vi "UWB_Controller.vi"() -> ()   [LabVIEW 2016]
doc: "This VI controlls the DWM over UART. It starts of by resetting the DWM by sending a reset message over UART. It then starts sending CR messages to the DWM and poll for a response. When anything is received on the poll the DWM is operational. It then starts to request a position message which it saves in a global variable later used by the ROS publisher."
uses:
  <vilib>/myRIO/Instrument Drivers/Onboard IO/UART/typedef/VISA Configuration.ctl
  <vilib>/myRIO/Instrument Drivers/Onboard IO/DIO/typedefs/DIO Reference.ctl
  <vilib>/myRIO/Common/Instrument Driver Framework/Utilities/typedefs/myRIO Generic Hardware Reference.ctl
  <vilib>/myRIO/Common/Instrument Driver Framework/Utilities/typedefs/Hardware Version Enum.ctl
  <vilib>/myRIO/Common/Instrument Driver Framework/Utilities/typedefs/myRIO v1.0 Reference.ctl
  <vilib>/myRIO/Common/Instrument Driver Framework/Utilities/typedefs/Generic FPGA Reference.ctl
  <vilib>/myRIO/Common/Instrument Driver Framework/myRIO v1.0/DIO/typedefs/DIO Channels List.ctl
  <vilib>/myRIO/Common/Instrument Driver Framework/myRIO v1.0/DIO/typedefs/DIO Channels Enum.ctl
  <vilib>/userdefined/High Color/nirio_resource_hc.ctl
  <vilib>/myRIO/Common/Instrument Driver Framework/Utilities/vis/Is FPGA Ref Available.vi
  <vilib>/myRIO/Common/Instrument Driver Framework/roboRIO v1.0/DIO/vis/roboRIO v1.0 Open DIO.vi
  <vilib>/myRIO/Instrument Drivers/Onboard IO/DIO/vis/Write.vi
  <vilib>/myRIO/Common/Instrument Driver Framework/Utilities/vis/Validate Channels.vi
  <vilib>/myRIO/Common/Instrument Driver Framework/roboRIO v1.0/DIO/vis/roboRIO v1.0 Reserve DIO.vi
  <vilib>/myRIO/Common/Instrument Driver Framework/roboRIO v1.0/DIO/vis/roboRIO v1.0 Build MUX Configuration DIO.vi
  <vilib>/myRIO/Common/Instrument Driver Framework/roboRIO v1.0/Resource Manager/vis/roboRIO v1.0 Reserve Channel List.vi
  <vilib>/myRIO/Common/Instrument Driver Framework/roboRIO v1.0/Resource Manager/vis/roboRIO v1.0 Create Configuration List.vi
  <vilib>/myRIO/Common/Instrument Driver Framework/roboRIO v1.0/Resource Manager/vis/roboRIO v1.0 Reserve Channel.vi
  <vilib>/myRIO/Common/Instrument Driver Framework/roboRIO v1.0/Resource Manager/vis/roboRIO v1.0 Unreserve Channel.vi
  <vilib>/myRIO/Common/Instrument Driver Framework/roboRIO v1.0/Resource Manager/vis/roboRIO v1.0 Build Mutex Name.vi
  <vilib>/Instr/_visa.llb/VISA Configure Serial Port (Instr).vi
  GlobalVI.vi
  <vilib>/Utility/VariantDataType/GetNumericInfo.vi
  builds/UnicornMain/UnicornRIO1/ROS for LabVIEW/home/lvuser/natinst/bin/vi.lib/Utility/error.llb/Error Cluster From Error Code.vi
  <vilib>/myRIO/Common/Instrument Driver Framework/roboRIO v1.0/roboRIO v1.0 Open.vi
  <vilib>/myRIO/Common/Instrument Driver Framework/Utilities/vis/IO Manager.vi
  <vilib>/myRIO/Common/Instrument Driver Framework/Utilities/vis/Configuration Manager.vi
  <vilib>/myRIO/Common/Instrument Driver Framework/roboRIO v1.0/Resource Manager/vis/roboRIO v1.0 Configure IO.vi
  <vilib>/myRIO/Common/Instrument Driver Framework/myRIO v1.0/myRIO v1.0 Close.vi
  <vilib>/myRIO/Common/Instrument Driver Framework/roboRIO v1.0/DIO/vis/roboRIO v1.0 Write DIO.vi
  <vilib>/myRIO/Express VI/Onboard IO/UART/UART Express VI.xnode
  <vilib>/regexp/Match Regular Expression.xnode
  <vilib>/myRIO/Express VI/Onboard Devices/LED/LED Express VI.xnode
  <vilib>/myRIO/Instrument Drivers/Onboard IO/DIO/vis/myRIO DIO Open.xnode
  <vilib>/myRIO/Instrument Drivers/Onboard IO/UART/UART.lvlib
  <vilib>/myRIO/Instrument Drivers/Onboard IO/DIO/DIO.lvlib
panel:
  out "error out":errorcluster
  in  "error in OUTPUT 3":errorcluster
  in  "error in INPUT 2":errorcluster
  out "currentTimeout_Receive":u32
  out "error out OUTPUT 2":errorcluster
  out "offset past match\n(-1 = no match)":i32
  out "MSGFound":bool
  out "X":dbl
  out "Y":dbl
  out "Z":dbl
  out "error out INPUT":errorcluster
  out "timeoutError":bool
  out "currentTimeout":u32
  out "timeoutCount":u32
  out "timeoutValue":u32
  out "Resetting...":bool
  out "System ON":bool
  out "Receiving":bool
  out "Transmitting":bool
  out "UART Reset Buffer":string
  out "uwbState":i32
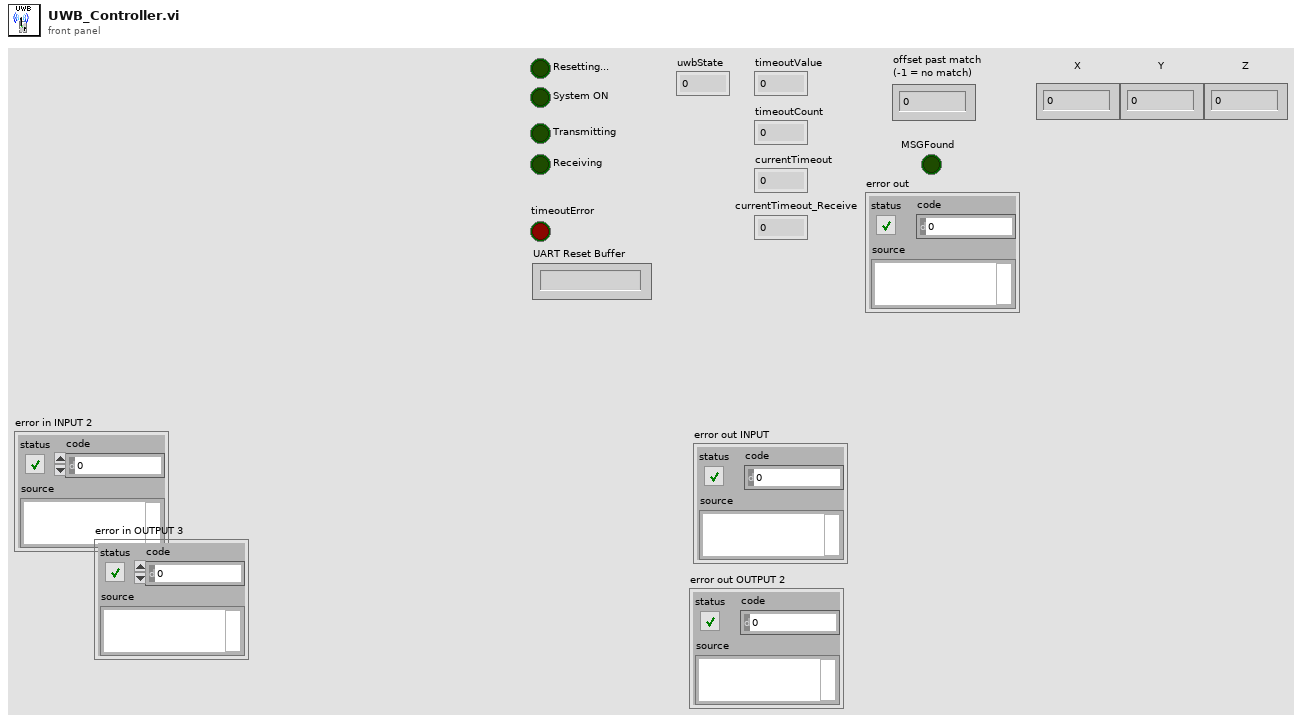
[diagram p1: front panel]
types:
  T1 = typedef "UART.lvlib/VISA Configuration.ctl" = cluster{"baud rate (9600)":u32, "data bits (8)":u16, "parity (0:none)":enum16{"None", "Odd", "Even", "Mark", "Space"}, "stop bits (10: 1 bit)":u16, "flow control (0:none)":u16, "termination char\n(0xA = '\\n' = LF) ":u8, "Enable Termination\nChar (T)":bool, "timeout (10sec)":u32}
  T2 = typedef "DIO.lvlib/DIO Reference.ctl" = cluster{"myRIO Reference":T3, "DIO Channels List":T7}
  T3 = typedef "myRIO Generic Hardware Reference.ctl" = cluster{"myRIO Model":T4, "myRIO Hardware Reference":T5}
  T4 = typedef "Hardware Version Enum.ctl" = enum16{"Unknown", "myRIO-1900", "myRIO-1950", "roboRIO", "NI ELVIS RIO CM"}
  T5 = typedef "myRIO v1.0 Reference.ctl" = cluster{"Generic FPGA Reference":T6, "Allow multiple opens":bool}
  T6 = typedef "Generic FPGA Reference.ctl" = refnum<k20>
  T7 = typedef "DIO Channels List.ctl" = T8[]
  T8 = typedef "DIO Channels Enum.ctl" = enum16{"Not Connected", "C/DIO0", "C/DIO1", "C/DIO2", "C/DIO3", "C/DIO4", "C/DIO5", "C/DIO6", "C/DIO7", "A/DIO0", "A/DIO1", "A/DIO2", "A/DIO3", "A/DIO4", "A/DIO5", "A/DIO6", "A/DIO7", "A/DIO8", "A/DIO9", "A/DIO10", "A/DIO11", "A/DIO12", "A/DIO13", "A/DIO14", "A/DIO15", "B/DIO0", "B/DIO1", "B/DIO2", "B/DIO3", "B/DIO4", "B/DIO5", "B/DIO6", "B/DIO7", "B/DIO8", "B/DIO9", "B/DIO10", "B/DIO11", "B/DIO12", "B/DIO13", "B/DIO14", "B/DIO15", "LED0", "LED1", "LED2", "LED3", "Button0", "DIO/DIO0", "DIO/DIO1", "DIO/DIO2", "DIO/DIO3", "DIO/DIO4", "DIO/DIO5", "DIO/DIO6", "DIO/DIO7", "DIO/DIO8", "DIO/DIO9", "SPI/CS0", "SPI/CS1", "SPI/CS2", "SPI/CS3", "LED RADIO (Green)", "LED RADIO (Red)", "LED COMM (Green)", "LED COMM (Red)", "LED MODE (Green)", "LED MODE (Red)"}
  T9 = typedef "nirio_resource_hc.ctl" = tag
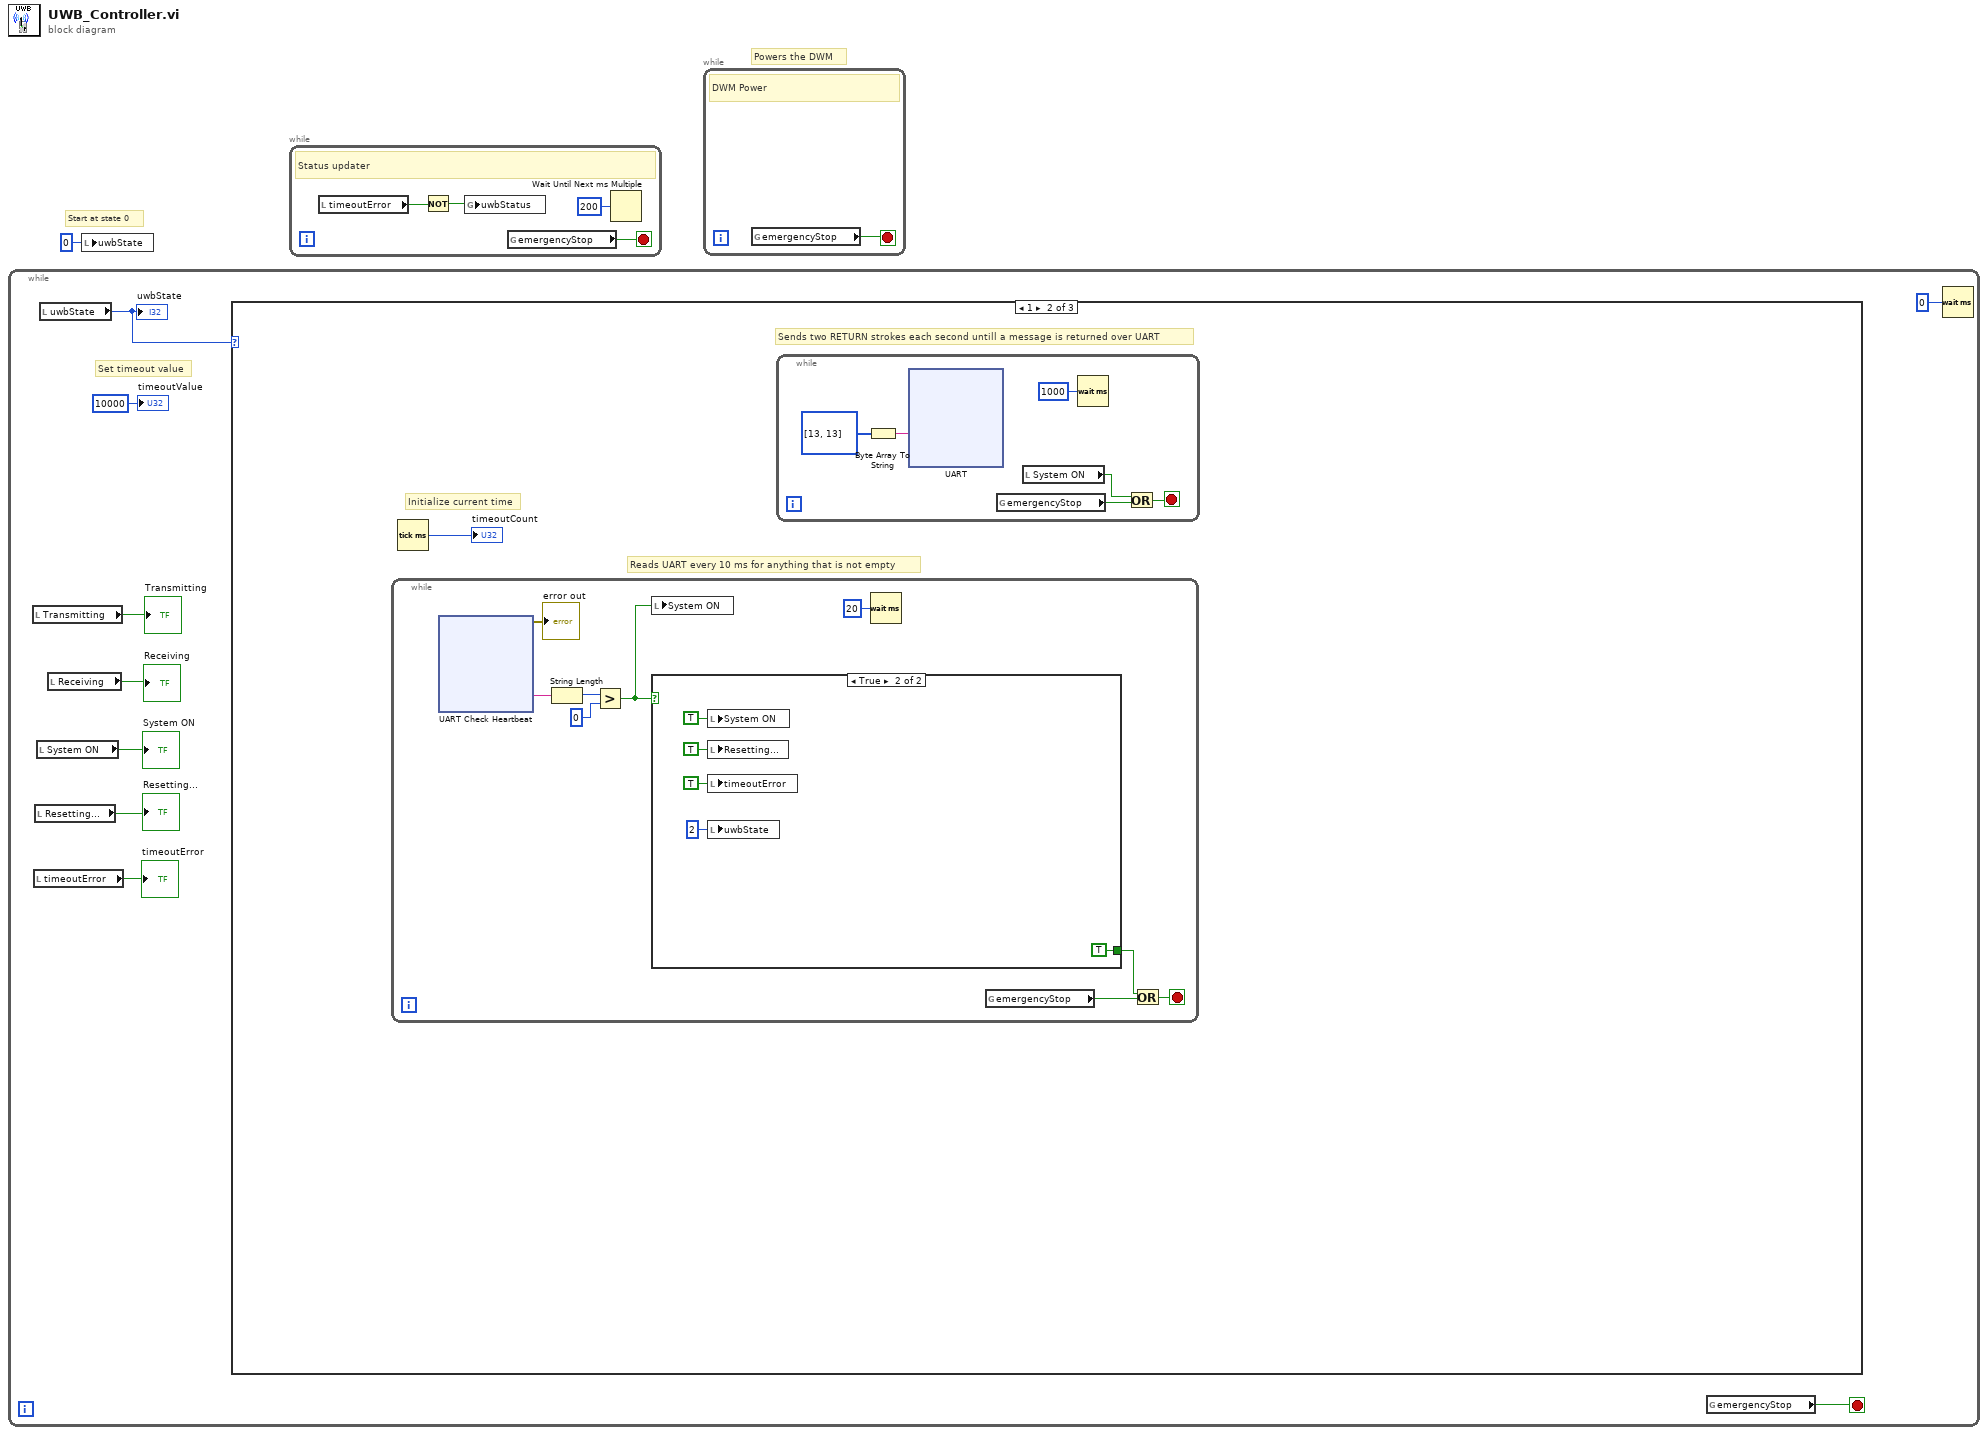
[diagram p0: block diagram]
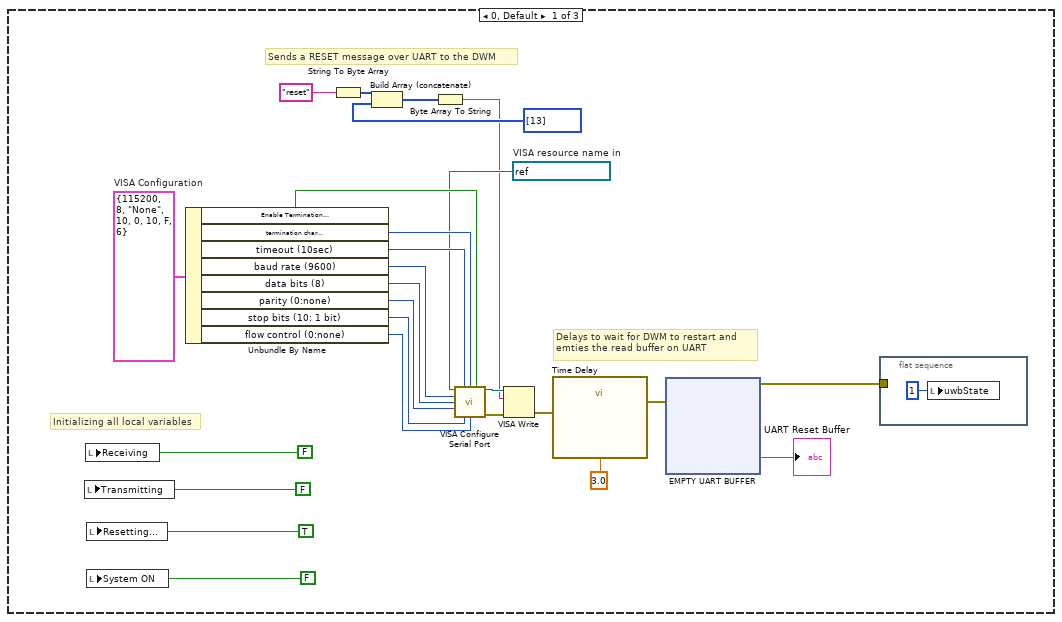
[diagram p2: hidden frame]
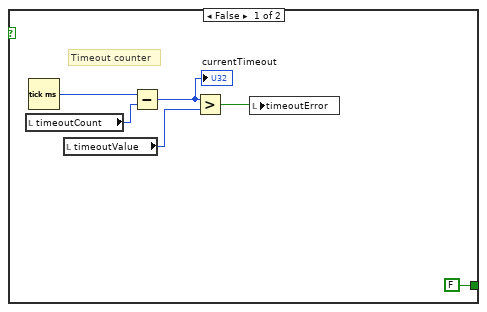
[diagram p3: hidden frame]
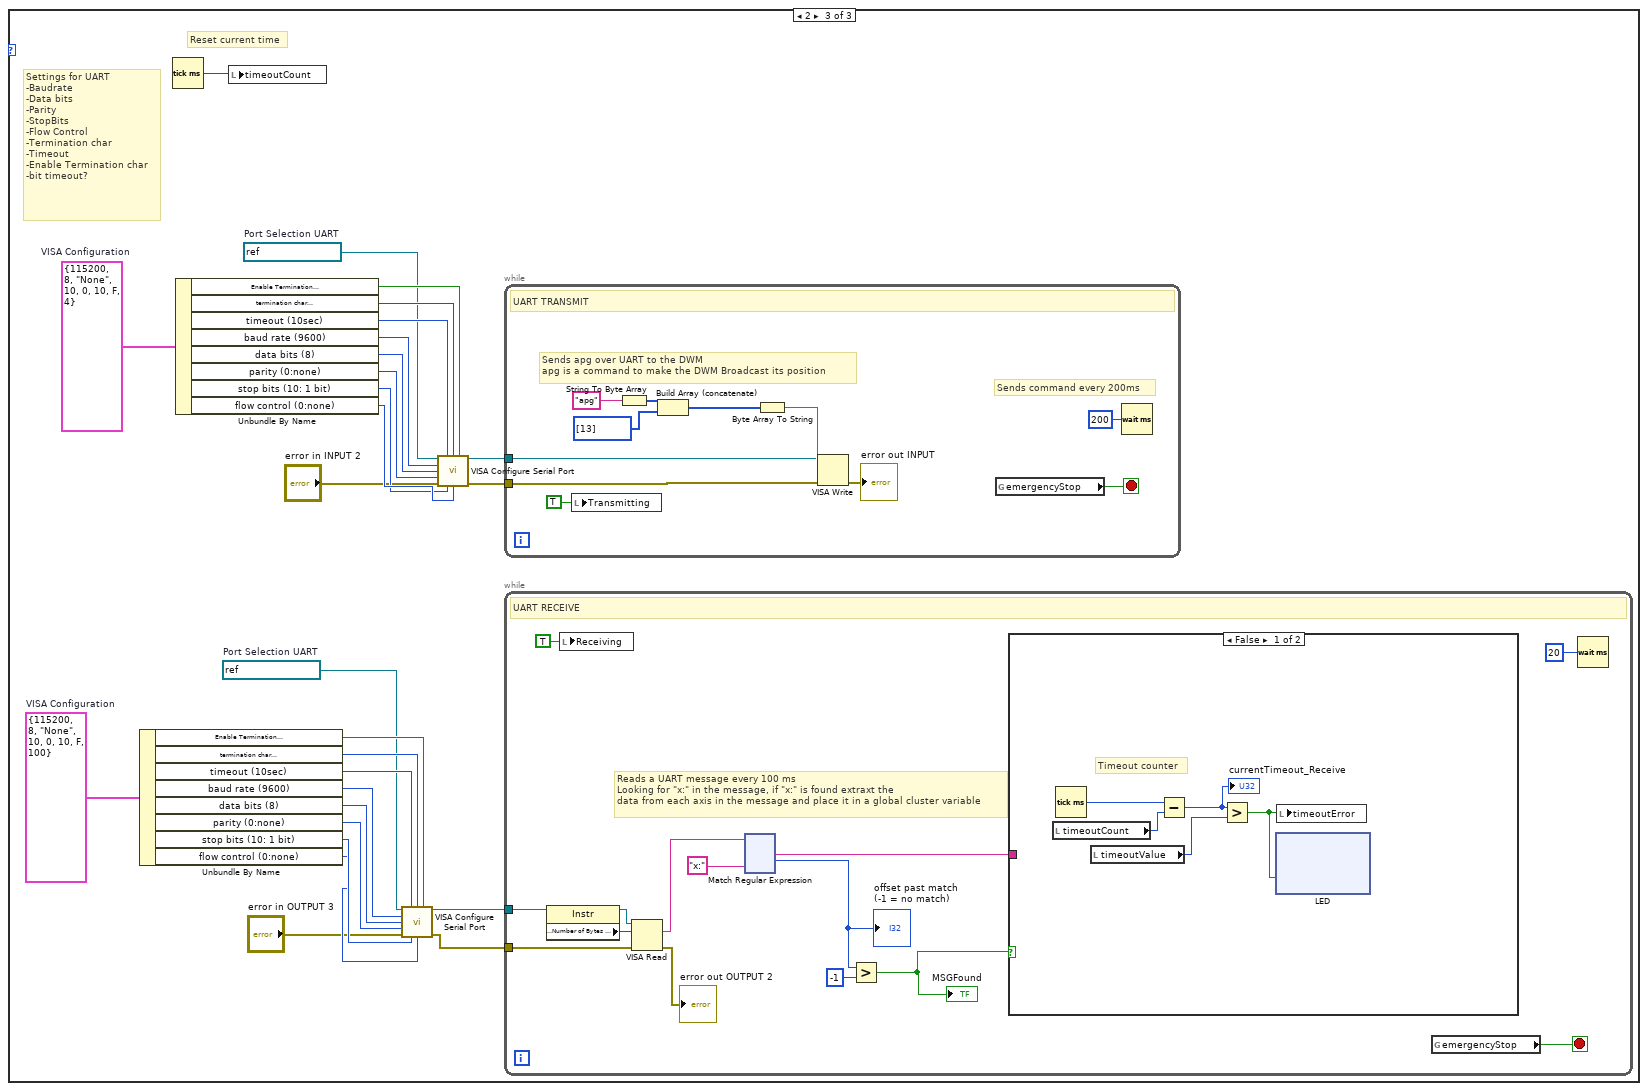
[diagram p4: hidden frame]
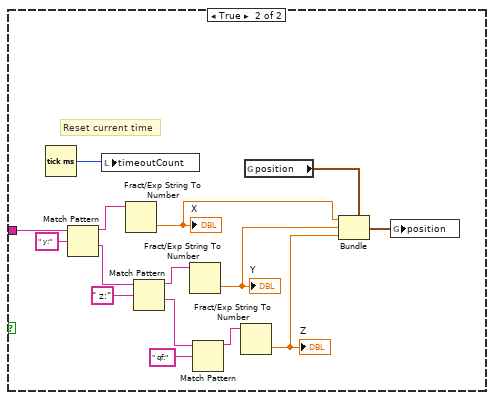
[diagram p5: hidden frame]
diagram:
  # "Powers the DWM"
  # "Start at state 0"
  n1 = while {
    stop <- w6 stop-if-true
    # "Set timeout value"
    n2 = local read "Transmitting"() -> (→"Transmitting":bool)
    n3 = local read "timeoutError"() -> (→"timeoutError":bool)
    n4 = local read "Resetting..."() -> (→"Resetting...":bool)
    n5 = local read "System ON"() -> (→"System ON":bool)
    n6 = local read "uwbState"() -> (w4:i32)
    "uwbState" <- w4
    n7 = local read "Receiving"() -> (→"Receiving":bool)
    n8 = case shown="1" w4 {
      frame 0, Default {
        w24 = T1 {"baud rate (9600)"=115200, "data bits (8)"=8, "parity (0:none)"=enum."None", "stop bits (10: 1 bit)"=10, "flow control (0:none)"=0, "termination char\n(0xA = '\\n' = LF) "=10, "Enable Termination\nChar (T)"=FALSE, "timeout (10sec)"=6}  # VISA Configuration
        w23 = refnum<visa-resource-name> "ASRL2::INSTR"  # VISA resource name in
        # "Initializing all local variables"
        # "Delays to wait for DWM to restart and \nemties the read buffer on UART"
        # "Sends a RESET message over UART to the DWM"
        n9 = local write "Transmitting"(FALSE ("Transmitting")) -> ()
        n10 = local write "Receiving"(FALSE ("Receiving")) -> ()
        n11 = local write "Resetting..."(TRUE ("Resetting...")) -> ()
        n12 = local write "System ON"(FALSE ("System On")) -> ()
        n13 = Unbundle By Name(w24) -> ("Enable Termination\nChar (T)"=w27:bool, "termination char\n(0xA = '\\n' = LF)"=w28:u8, "timeout (10sec)"=w29:u32, "baud rate (9600)"=w34:u32, "data bits (8)"=w33:u16, "parity (0:none)"=w32:enum16{"None", "Odd", "Even", "Mark", "Space"}, "stop bits (10: 1 bit)"=w31:u16, "flow control (0:none)"=w30:u16)
        n14 = String To Byte Array(string="reset") -> (unsigned byte array=w19:u8[])
        n15 = Build Array (concatenate)(w19, i32[] [13]) -> (w18:i32[])
        n16 = Byte Array To String(unsigned byte array=w18) -> (string=w17:string)
        n17 = call-poly "VISA Configure Serial Port"("VISA resource name"=w23, "timeout (10sec)"=w29, "termination char\n(0xA = '\\n' = LF)"=w28, "Enable Termination\nChar (T)"=w27, "baud rate (9600)"=w34, "data bits (8)"=w33, "parity (0:none)"=w32, "stop bits (10: 1 bit)"=w31, "flow control (0:none)"=w30) -> ("VISA resource name out"=w25:refnum<visa-resource-name>, "error out"=w26:errorcluster)  [unwired: 5 in]
        n18 = VISA Write(VISA resource name=w25, write buffer=w17, error in (no error)=w26) -> (error out=w22:errorcluster)  [unwired: 2 out]
        n19 = call "Time Delay"("error in (no error)"=w22, "Delay Time (s)"=3.0) -> ("error out"=w35:errorcluster)  [unwired: 9 in]
        n20 = xnode "EMPTY UART BUFFER"("error in (no error)"=w35) -> ("Characters Read"=→"UART Reset Buffer":string, "error out"=w11:errorcluster)
        n21 = flat-sequence {
          tunnel: w11 -> [_]
          frame #0 {
            n22 = local write "uwbState"(1 ("uwbState")) -> ()
          }
        }
      }
      frame 1 {
        # "Initialize current time"
        # "Reads UART every 10 ms for anything that is not empty"
        # "Sends two RETURN strokes each second untill a message is returned over UART"
        n23 = while {
          stop <- w81 stop-if-true
          n24 = xnode "UART Check Heartbeat"() -> ("Characters Read"=w86:string, "error out"=→"error out":errorcluster)  [unwired: 1 in]
          n25 = String Length(string=w86) -> (length=w85:i32)
          n26 = Greater?(x=w85, y=0) -> (0:w82:bool)
          n27 = local write "System ON"(w82) -> ()
          n28 = case shown="True" w82 {
            tunnel: [FALSE TRUE] -> w80
            frame False {
              # "Timeout counter"
              n29 = local read "timeoutCount"() -> (w89:u32)
              n30 = Tick Count (ms)() -> (millisecond timer value=w91:u32)
              n31 = local read "timeoutValue"() -> (w90:u32)
              n32 = Subtract(x=w91, y=w89) -> (x-y=w88:u32)
              "currentTimeout" <- w88
              n33 = Greater?(x=w88, y=w90) -> (0:w87:bool)
              n34 = local write "timeoutError"(w87) -> ()
            }
            frame True {
              n35 = local write "System ON"(TRUE ("System ON")) -> ()
              n36 = local write "Resetting..."(TRUE ("Resetting...")) -> ()
              n37 = local write "timeoutError"(TRUE ("timeoutError")) -> ()
              n38 = local write "uwbState"(2 ("uwbState")) -> ()
            }
          }
          n39 = Wait (ms)(milliseconds to wait=u32 20) -> ()  [unwired: 1 out]
          n40 = global read "GlobalVI.vi" "emergencyStop"() -> (w79:bool)
          n41 = Or(x=w80, y=w79) -> (x .or. y?=w81:bool)
        }
        n42 = Tick Count (ms)() -> (millisecond timer value=→"timeoutCount":u32)
        n43 = while {
          stop <- w57 stop-if-true
          n44 = Byte Array To String(unsigned byte array=u8[] [13, 13]) -> (string=w61:string)
          n45 = xnode "UART"("Characters to Write"=w61) -> ()  [unwired: 1 in, 2 out]
          n46 = global read "GlobalVI.vi" "emergencyStop"() -> (w58:bool)
          n47 = local read "System ON"() -> (w56:bool)
          n48 = Wait (ms)(milliseconds to wait=u32 1000) -> ()  [unwired: 1 out]
          n49 = Or(x=w56, y=w58) -> (x .or. y?=w57:bool)
        }
      }
      frame 2 {
        w118 = T1 {"baud rate (9600)"=115200, "data bits (8)"=8, "parity (0:none)"=enum."None", "stop bits (10: 1 bit)"=10, "flow control (0:none)"=0, "termination char\n(0xA = '\\n' = LF) "=10, "Enable Termination\nChar (T)"=FALSE, "timeout (10sec)"=100}  # VISA Configuration
        w117 = refnum<visa-resource-name> "ASRL2::INSTR"  # Port Selection UART
        w131 = T1 {"baud rate (9600)"=115200, "data bits (8)"=8, "parity (0:none)"=enum."None", "stop bits (10: 1 bit)"=10, "flow control (0:none)"=0, "termination char\n(0xA = '\\n' = LF) "=10, "Enable Termination\nChar (T)"=FALSE, "timeout (10sec)"=4}  # VISA Configuration
        w130 = refnum<visa-resource-name> "ASRL2::INSTR"  # Port Selection UART
        # "Settings for UART\n-Baudrate\n-Data bits\n-Parity\n-StopBits\n-Flow Control\n-Termination char\n-Timeout\n-Enable Termination char\n-bit timeout?"
        # "Reset current time"
        n50 = Unbundle By Name(w118) -> ("Enable Termination\nChar (T)"=w120:bool, "termination char\n(0xA = '\\n' = LF)"=w121:u8, "timeout (10sec)"=w122:u32, "baud rate (9600)"=w127:u32, "data bits (8)"=w126:u16, "parity (0:none)"=w125:enum16{"None", "Odd", "Even", "Mark", "Space"}, "stop bits (10: 1 bit)"=w124:u16, "flow control (0:none)"=w123:u16)
        n51 = Tick Count (ms)() -> (millisecond timer value=w141:u32)
        n52 = Unbundle By Name(w131) -> ("Enable Termination\nChar (T)"=w133:bool, "termination char\n(0xA = '\\n' = LF)"=w134:u8, "timeout (10sec)"=w135:u32, "baud rate (9600)"=w139:u32, "data bits (8)"=w138:u16, "parity (0:none)"=w137:enum16{"None", "Odd", "Even", "Mark", "Space"}, "stop bits (10: 1 bit)"=w136:u16, "flow control (0:none)"=w140:u16)
        n53 = local write "timeoutCount"(w141) -> ()
        n54 = call-poly "VISA Configure Serial Port"("VISA resource name"=w117, "timeout (10sec)"=w122, "termination char\n(0xA = '\\n' = LF)"=w121, "Enable Termination\nChar (T)"=w120, "baud rate (9600)"=w127, "data bits (8)"=w126, "parity (0:none)"=w125, "error in (no error)"="error in OUTPUT 3", "stop bits (10: 1 bit)"=w124, "flow control (0:none)"=w123) -> ("VISA resource name out"=w116:refnum<visa-resource-name>, "error out"=w115:errorcluster)  [unwired: 4 in]
        n55 = call-poly "VISA Configure Serial Port"("VISA resource name"=w130, "timeout (10sec)"=w135, "termination char\n(0xA = '\\n' = LF)"=w134, "Enable Termination\nChar (T)"=w133, "baud rate (9600)"=w139, "data bits (8)"=w138, "parity (0:none)"=w137, "error in (no error)"="error in INPUT 2", "stop bits (10: 1 bit)"=w136, "flow control (0:none)"=w140) -> ("VISA resource name out"=w129:refnum<visa-resource-name>, "error out"=w128:errorcluster)  [unwired: 4 in]
        n56 = while {
          tunnel: w129 -> [w326]
          tunnel: w128 -> [w325]
          stop <- w327 stop-if-true
          # "Sends command every 200ms"
          # "Sends apg over UART to the DWM\napg is a command to make the DWM Broadcast its position"
          # "UART TRANSMIT"
          n57 = local write "Transmitting"(TRUE ("Transmitting")) -> ()
          n58 = String To Byte Array(string="apg") -> (unsigned byte array=w332:u8[])
          n59 = Build Array (concatenate)(w332, i32[] [13]) -> (w331:i32[])
          n60 = Byte Array To String(unsigned byte array=w331) -> (string=w335:string)
          n61 = VISA Write(VISA resource name=w326, write buffer=w335, error in (no error)=w325) -> (error out=→"error out INPUT":errorcluster)  [unwired: 2 out]
          n62 = global read "GlobalVI.vi" "emergencyStop"() -> (w327:bool)
          n63 = Wait (ms)(milliseconds to wait=u32 200) -> ()  [unwired: 1 out]
        }
        n64 = while {
          tunnel: w116 -> [w143]
          tunnel: w115 -> [w142]
          stop <- w144 stop-if-true
          # "Reads a UART message every 100 ms\nLooking for \"x:\" in the message, if \"x:\" is found extraxt the\ndata from each axis in the message and place it in a global cluster variable"
          # "UART RECEIVE"
          n65 = property class="Instr"(reference=w143) -> (reference out=w153:refnum<visa-resource-name>, "Serial Settings:Number of Bytes at Serial Port"=w154:u32)  [unwired: 1 in, 1 out]
          n66 = local write "Receiving"(TRUE ("Receiving")) -> ()
          n67 = VISA Read(VISA resource name=w153, byte count=w154, error in (no error)=w142) -> (read buffer=w147:string, error out=→"error out OUTPUT 2":errorcluster)  [unwired: 2 out]
          n68 = xnode "Match Regular Expression"("input string"=w147, "regular expression"="x:") -> ("after match"=w146:string, "offset past match"=w150:i32)  [unwired: 4 in, 3 out]
          "offset past match\n(-1 = no match)" <- w150
          n69 = Greater?(x=w150, y=-1) -> (0:w148:bool)
          "MSGFound" <- w148
          n70 = case shown="False" w148 {
            tunnel: w146 -> [_ w202]
            frame False {
              # "Timeout counter"
              n71 = local read "timeoutCount"() -> (w158:u32)
              n72 = Tick Count (ms)() -> (millisecond timer value=w160:u32)
              n73 = local read "timeoutValue"() -> (w159:u32)
              n74 = Subtract(x=w160, y=w158) -> (x-y=w157:u32)
              "currentTimeout_Receive" <- w157
              n75 = Greater?(x=w157, y=w159) -> (0:w156:bool)
              n76 = xnode "LED"("RADIO (Red)"=w156) -> ()  [unwired: 1 in, 1 out]
              n77 = local write "timeoutError"(w156) -> ()
            }
            frame True {
              # "Reset current time"
              n78 = Tick Count (ms)() -> (millisecond timer value=w197:u32)
              n79 = Match Pattern(string=w202, regular expression=" y:") -> (before substring=w209:string, after substring=w208:string)  [unwired: 1 in, 2 out]
              n80 = local write "timeoutCount"(w197) -> ()
              n81 = Fract/Exp String To Number(string=w209) -> (number=w200:dbl)  [unwired: 3 in, 1 out]
              "X" <- w200
              n82 = Match Pattern(string=w208, regular expression=" z:") -> (before substring=w206:string, after substring=w207:string)  [unwired: 1 in, 2 out]
              n83 = Fract/Exp String To Number(string=w206) -> (number=w199:dbl)  [unwired: 3 in, 1 out]
              "Y" <- w199
              n84 = Match Pattern(string=w207, regular expression=" qf:") -> (before substring=w205:string)  [unwired: 1 in, 3 out]
              n85 = Fract/Exp String To Number(string=w205) -> (number=w198:dbl)  [unwired: 3 in, 1 out]
              "Z" <- w198
              n86 = global read "GlobalVI.vi" "position"() -> (w201:cluster{"x":dbl, "y":dbl, "z":dbl})
              n87 = Bundle(cluster=w201, "x"=w200, "y"=w199, "z"=w198) -> (w196:cluster{"x":dbl, "y":dbl, "z":dbl})
              n88 = global write "GlobalVI.vi" "position"(w196) -> ()
            }
          }
          n89 = global read "GlobalVI.vi" "emergencyStop"() -> (w144:bool)
          n90 = Wait (ms)(milliseconds to wait=u32 20) -> ()  [unwired: 1 out]
        }
      }
    }
    n91 = global read "GlobalVI.vi" "emergencyStop"() -> (w6:bool)
    n92 = Wait (ms)(milliseconds to wait=u32 0) -> ()  [unwired: 1 out]
    "timeoutValue" <- u32 10000 ("timeoutValue")
  }
  n93 = local write "uwbState"(0 ("uwbState")) -> ()
  n94 = while {
    stop <- w339 stop-if-true
    # "Status updater"
    n95 = local read "timeoutError"() -> (w338:bool)
    n96 = Not(x=w338) -> (.not. x?=w337:bool)
    n97 = global write "GlobalVI.vi" "uwbStatus"(w337) -> ()
    n98 = global read "GlobalVI.vi" "emergencyStop"() -> (w339:bool)
    n99 = Wait Until Next ms Multiple(millisecond multiple=u32 200) -> ()  [unwired: 1 out]
  }
  n100 = while {
    stop <- w340 stop-if-true
    # "DWM Power"
    n101 = global read "GlobalVI.vi" "emergencyStop"() -> (w340:bool)
  }
